vi "Query.vi"(0 "VISA resource name":refnum<visa-resource-name>, 5 "error in (no error)":errorcluster) -> (15 "Array 3":T1[](array[typedef]), 19 "error out":errorcluster)   [LabVIEW 2016]
uses:
  Controls/Control System Visa Address and String cluster.ctl
panel:
  out "VISA resource name out":refnum<visa-resource-name>
  out "Array 2":i32[](array[numeric])
  out "Array":string[](array[string])
  out "return count":u32
  out "read buffer":string
  out "length":i32
  out "Numeric Control":i32
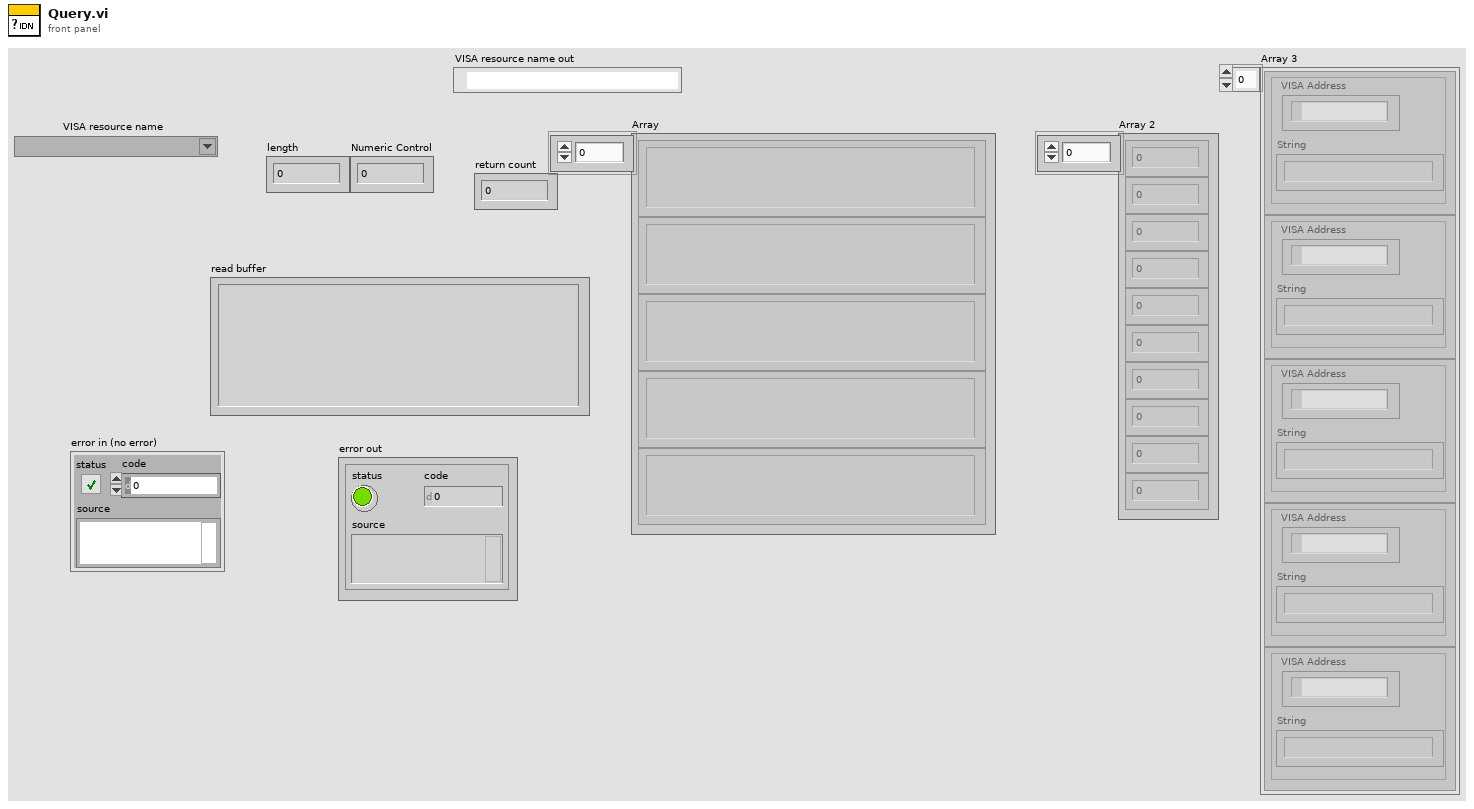
[diagram p1: front panel]
types:
  T1 = typedef "Control System Visa Address and String cluster.ctl" = cluster{"VISA Address":refnum<visa-resource-name>, "String":string}
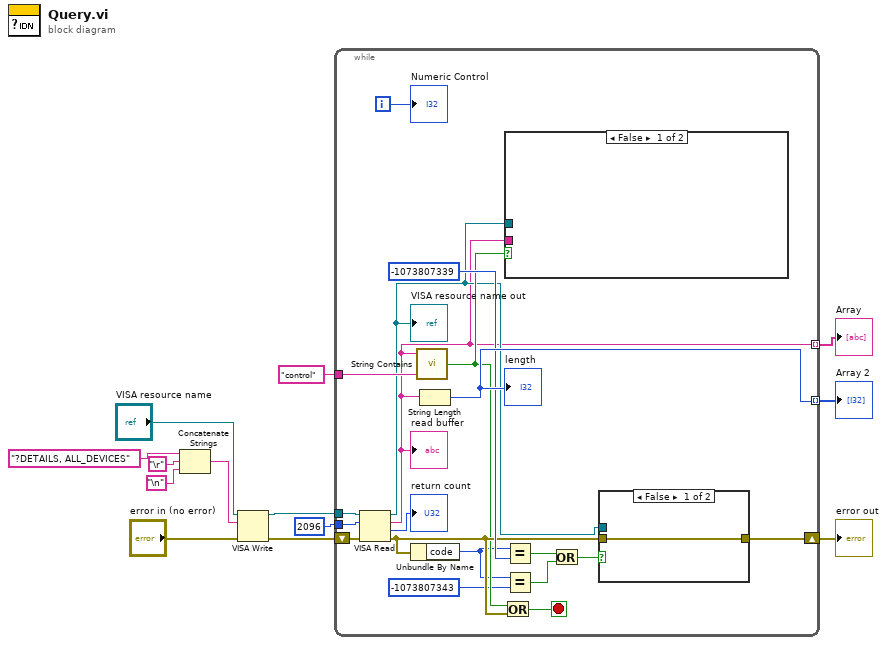
[diagram p0: block diagram]
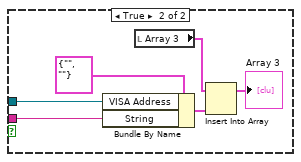
[diagram p2: hidden frame]
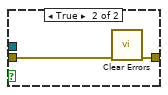
[diagram p3: hidden frame]
diagram:
  n1 = Concatenate Strings("?DETAILS, ALL_DEVICES" ("string"), "\r", "\n") -> (w10:string)
  n2 = VISA Write(VISA resource name="VISA resource name", write buffer=w10, error in (no error)="error in (no error)") -> (VISA resource name out=w13:refnum<visa-resource-name>, error out=w12:errorcluster)  [unwired: 1 out]
  n3 = while {
    shift-right: [w24] -> w11
    shift-left: w12 -> [w31]
    tunnel: u32 2096 ("byte count") -> [w28]
    tunnel: [w26] -> w4 mode=indexing
    tunnel: w13 -> [w32]
    tunnel: "control" -> [w22]
    tunnel: [w19] -> w1 mode=indexing
    i -> [w29]
    stop <- w27 stop-if-true
    n4 = VISA Read(VISA resource name=w32, byte count=w28, error in (no error)=w31) -> (VISA resource name out=w20:refnum<visa-resource-name>, read buffer=w19:string, return count=→"return count":u32, error out=w23:errorcluster)
    "read buffer" <- w19
    "VISA resource name out" <- w20
    n5 = Unbundle By Name(w23) -> ("code"=w18:i32)
    n6 = call "String Contains.vi"("Regular expression"=w22, "Input String"=w19) -> ("Found?"=w21:bool)  [unwired: 2 in, 1 out]
    n7 = String Length(string=w19) -> (length=w26:i32)
    "length" <- w26
    n8 = Or(x=w21, y=w23) -> (x .or. y?=w27:bool)
    n9 = case shown="False" w21 {
      tunnel: w20 -> [_ w37]
      tunnel: w19 -> [_ w36]
      frame False {
      }
      frame True {
        n10 = Bundle By Name(cluster=T1 {"VISA Address"="", "String"=""} ("Cluster"), "VISA Address"=w37, "String"=w36) -> (w35:T1)
        n11 = local read "Array 3"() -> (w33:T1[])
        n12 = Insert Into Array(array=w33, new element=w35) -> (→"Array 3":T1[])  [unwired: 1 in]
      }
    }
    n13 = Equal?(x=w18, y=-1073807339 ("code")) -> (x = y?=w16:bool)
    n14 = Equal?(x=w18, y=-1073807343) -> (x = y?=w15:bool)
    n15 = Or(x=w16, y=w15) -> (x .or. y?=w14:bool)
    n16 = case shown="False" w14 {
      tunnel: w23 -> [w39 w41]
      tunnel: [w39 w40] -> w24
      tunnel: w20 -> [_ _]
      frame False {
      }
      frame True {
        n17 = call <vilib>:"Clear Errors.vi"("error in (no error)"=w41) -> ("error out"=w40:errorcluster)  [unwired: 5 in, 1 out]
      }
    }
    "Numeric Control" <- w29
  }
  "error out" <- w11
  "Array" <- w1
  "Array 2" <- w4
